vi "Set 7Parameter DIO.vi"(8 "error in (no error)":errorcluster caption="entrée d'erreur (pas d'erreur)", 10 "Parameter":T1, 11 "Class Popup WaitDIO en entrée":refnum<class "Class Popup WaitShieldingBox.lvclass">) -> (0 "error out":errorcluster caption="sortie d'erreur", 3 "Class Popup WaitDIO en sortie":refnum<class "Class Popup WaitShieldingBox.lvclass">)   [LabVIEW 2020, in "Library Instrument & Equipement.lvlib" / "Library Popup.lvlib" / "Class Popup WaitShieldingBox.lvclass"]
uses:
  Class Popup WaitShieldingBox.lvclass
  Instrument/Instrument (Default)/Class Instrument (Default).lvclass
  Class Popup WaitShieldingBox.lvclass/Class Popup WaitShieldingBox.ctl
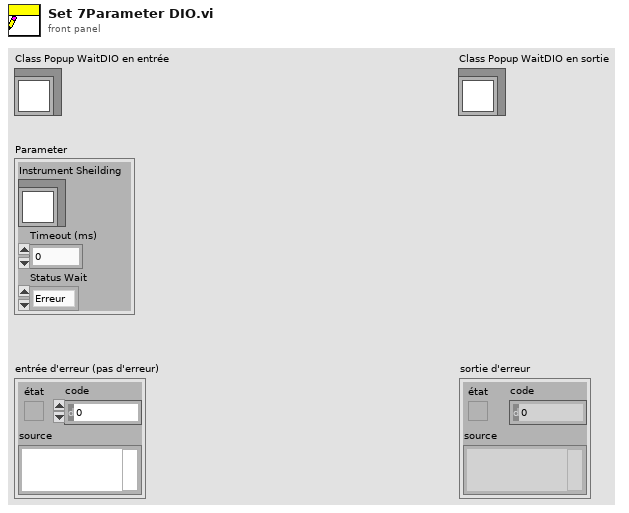
[diagram p1: front panel]
types:
  T1 = cluster{"Instrument Sheilding":refnum<class "Class Instrument (Default).lvclass">, "Timeout (ms)":u64, "Status Wait":enum16{"Erreur", "Close", "Open"}}
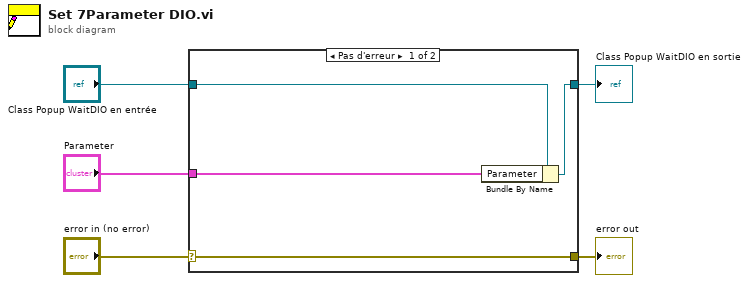
[diagram p0: block diagram]
diagram:
  n1 = case shown="Pas d'erreur" "error in (no error)" {
    selector: "error in (no error)" -> [w9 w10]
    tunnel: [w9 w10] -> w4
    tunnel: [w7 w11] -> w2
    tunnel: "Class Popup WaitDIO en entrée" -> [w8 w11]
    tunnel: "Parameter" -> [w6 _]
    frame No Error {
      n2 = Bundle By Name(cluster=w8, "Parameter"=w6) -> (w7:refnum<class "Class Popup WaitShieldingBox.lvclass">)
    }
    frame Error {
    }
  }
  "error out" <- w4
  "Class Popup WaitDIO en sortie" <- w2
